vi "CanChannelInitialize.vi"(4 "TX Fifo Size":u16, 5 "RX Fifo Size":u16, 6 "error in":errorcluster {"code" format="%.0x"}, 7 "TX Threshold":u16, 8 "RX Threshold":u16, 9 "CAN Channel Handle in":u32 format="%x") -> (0 "error out":errorcluster {"code" format="%.0x"}, 2 "Init OK":bool, 3 "CAN Channel Handle out":u32)   [LabVIEW 2012]
doc: "Initializes the CAN channel with the specified FIFO sizes and event trigger limits."
uses:
  vcilva.dll
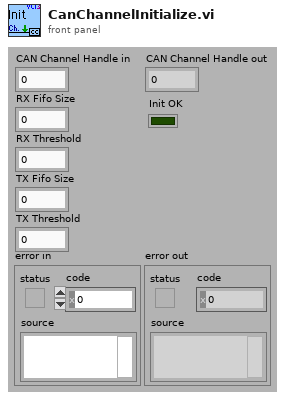
[diagram p1: front panel]
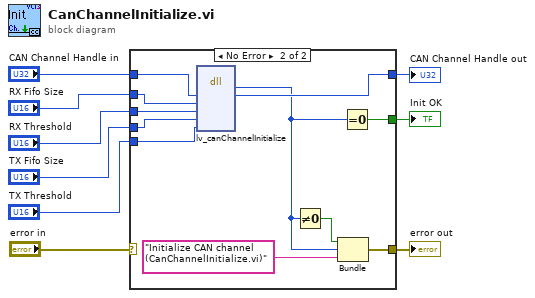
[diagram p0: block diagram]
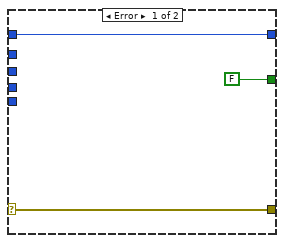
[diagram p2: hidden frame]
diagram:
  n1 = case shown="No Error" "error in" {
    selector: "error in" -> [w12 _]
    tunnel: [w12 w23] -> w8
    tunnel: "CAN Channel Handle in" -> [w11 w20]
    tunnel: [w11 w19] -> w6
    tunnel: "RX Fifo Size" -> [_ w18]
    tunnel: "RX Threshold" -> [_ w17]
    tunnel: "TX Fifo Size" -> [_ w16]
    tunnel: "TX Threshold" -> [_ w15]
    tunnel: [FALSE w14] -> w1
    frame Error {
    }
    frame No Error {
      n2 = dll-call lib="vcilva.dll" fn="lv_canChannelInitialize"("hCanChn"=w20, "wRxFifoSize"=w18, "wRxThreshold"=w17, "wTxFifoSize"=w16, "wTxThreshold"=w15) -> (w13:i32, "hCanChn"=w19:u32)  [unwired: 7 in, 2 out]
      n3 = Not Equal To 0?(x=w13) -> (x != 0?=w22:bool)
      n4 = Bundle(w22, w13, "Initialize CAN channel (CanChannelInitialize.vi)") -> (w23:errorcluster)  [unwired: 1 in]
      n5 = Equal To 0?(x=w13) -> (x = 0?=w14:bool)
    }
  }
  "error out" <- w8
  "CAN Channel Handle out" <- w6
  "Init OK" <- w1
